vi "Debug Cell Performance.vi"() -> ()   [LabVIEW 2021]
uses:
  Ethernet/Ethernet_BS1201.lvclass
  TypeDefs/System Status.ctl
  BS120x.lvclass
panel:
  in  "Cell to view":i32=1 min=1 max=12
  out "I pk-pk 2":dbl
  out "I read average 2":dbl
  out "V pk-pk 2":dbl
  out "V Read Average 2":dbl
  in  "Run":bool
  in  "Number of Samples":i32=1 min=1 max=12
  in  "Precision":bool
  in  "PID Disable":bool
  in  "Reset Unit":bool
  out "error out":errorcluster
  out "Cell Current":dbl[](array[numeric]) format="%#8.1f"
  out "Cell Voltages":dbl[](array[numeric])
  in  "Voltage Set All":dbl
  in  "Sink I All":dbl
  in  "Source I All":dbl
  out "Status":T1
  in  "Enable All Cells":bool
  in  "UDP port":u16=54321
  in  "TCP port":u16=12345
  in  "Box IP address":string="192.168.1.100"
  in  "stop":bool
  out "Voltages 2":dbl[](graph)
  out "Currents 2":dbl[](graph)
  # "(c) 2019 Bloomy Controls, Inc. All rights reserved."
  # "Cell Performance"
  # "Configuration"
  # "Write All Channels"
  # "Read"
  # "1"
  # "6"
  # "Operational Config"
  # "12"
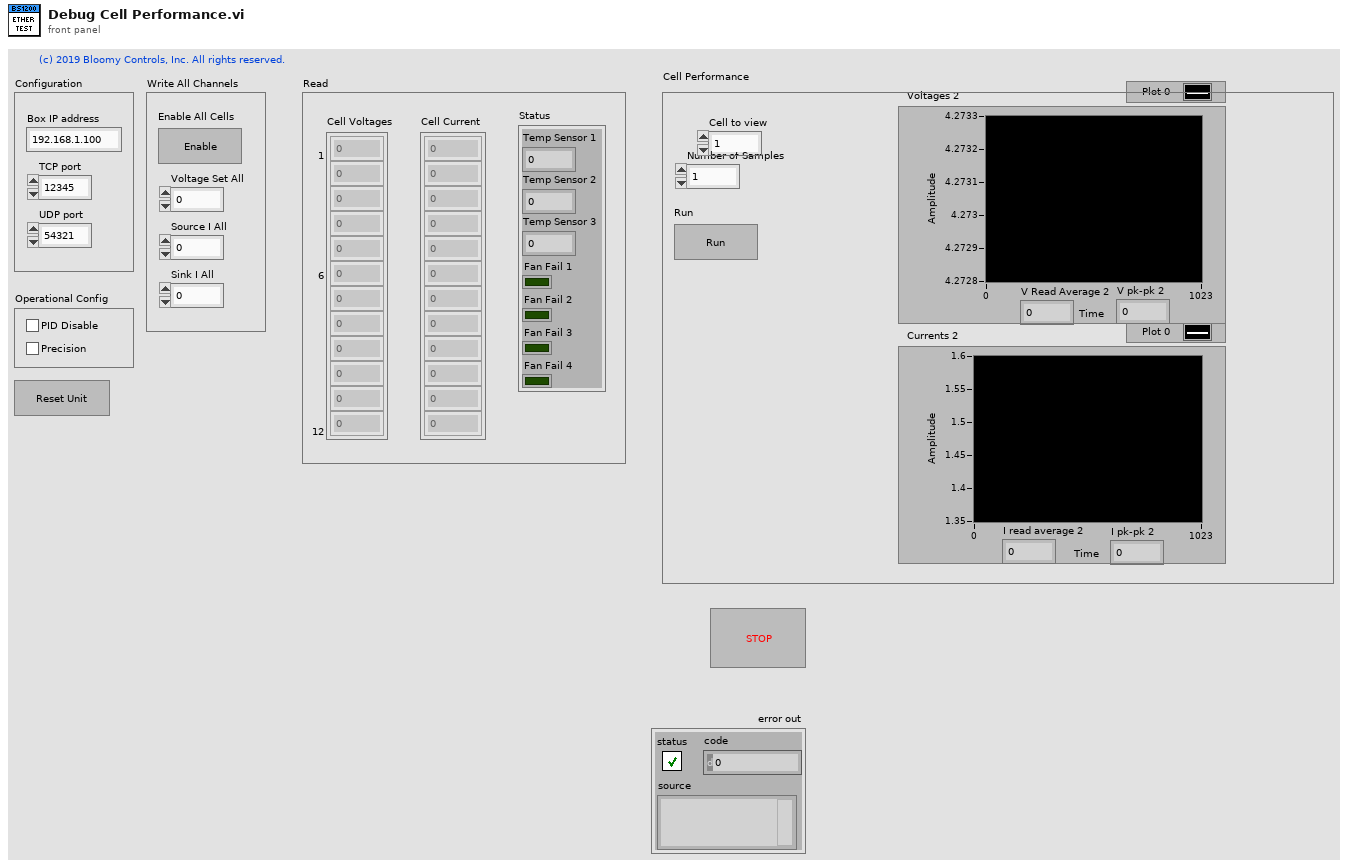
[diagram p1: front panel]
types:
  T1 = typedef "BS120x Driver.lvlib/BS120x.lvclass/System Status.ctl" = cluster{"Temp Sensor 1":dbl, "Temp Sensor 2":dbl, "Temp Sensor 3":dbl, "Fan Fail 1":bool, "Fan Fail 2":bool, "Fan Fail 3":bool, "Fan Fail 4":bool}
  T2 = typedef "Battery Simulator 1200 LabVIEW Driver.lvlib/Battery Simulator 1200 Driver.lvclass/System Status.ctl" = cluster{"Temp Sensor 1":dbl, "Temp Sensor 2":dbl, "Temp Sensor 3":dbl, "Fan Fail 1":bool, "Fan Fail 2":bool, "Fan Fail 3":bool, "Fan Fail 4":bool}
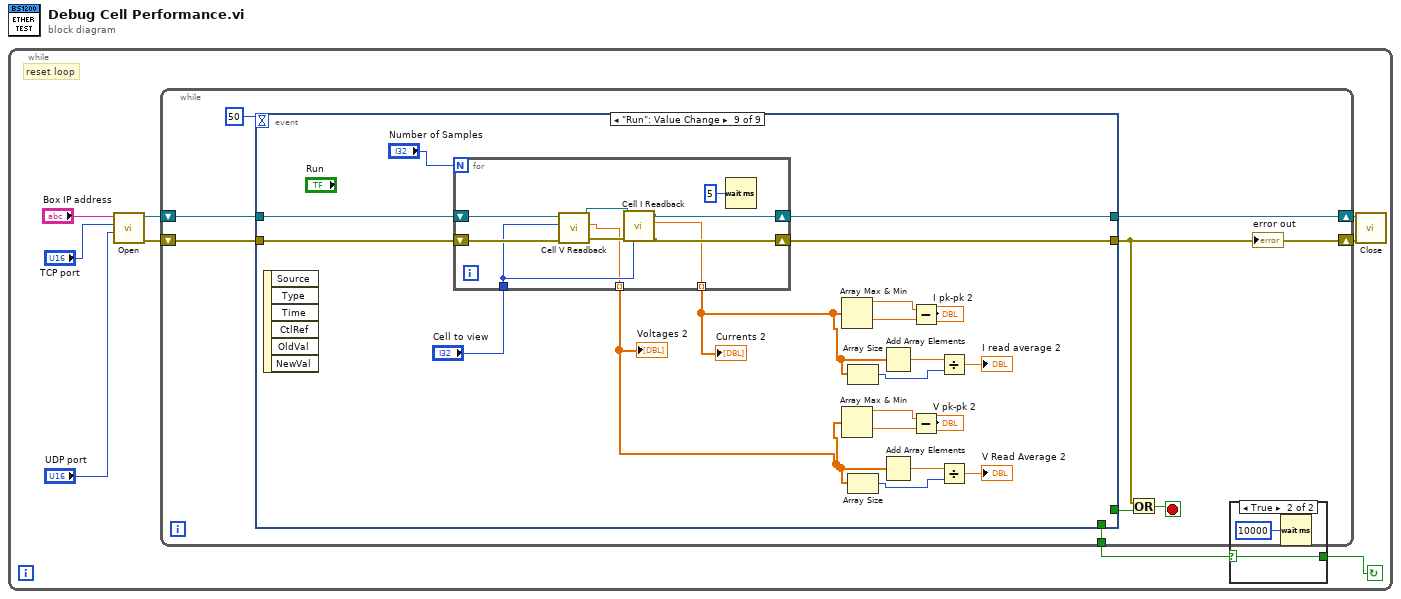
[diagram p0: block diagram]
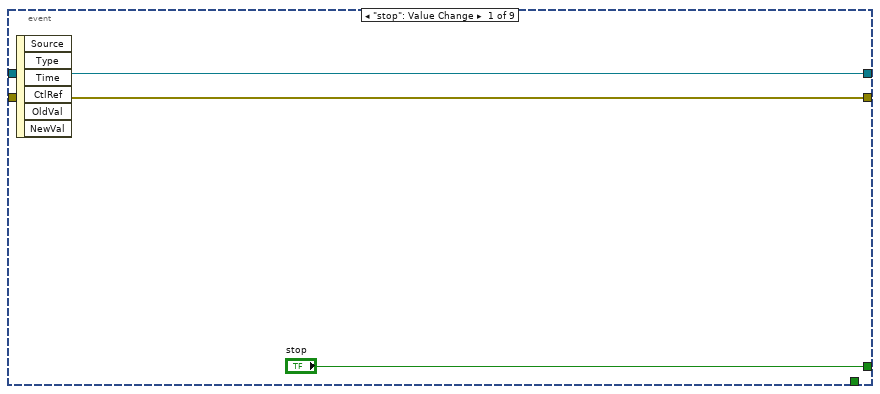
[diagram p3: hidden frame]
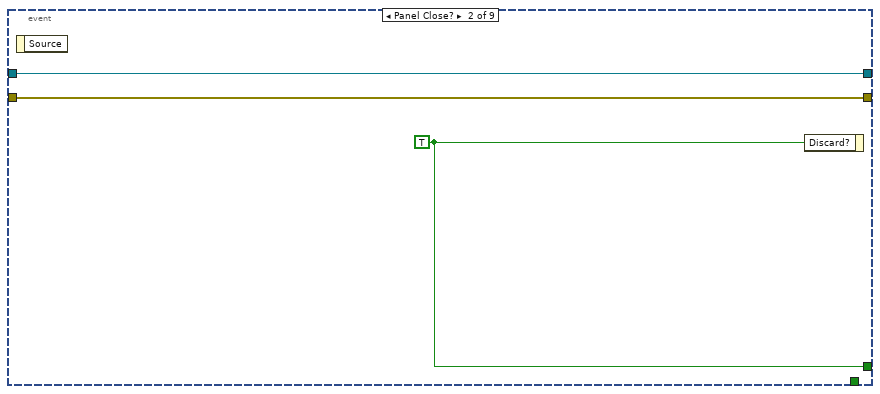
[diagram p4: hidden frame]
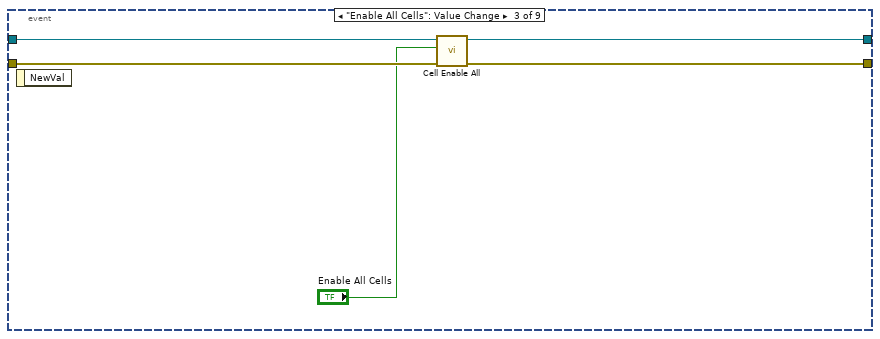
[diagram p5: hidden frame]
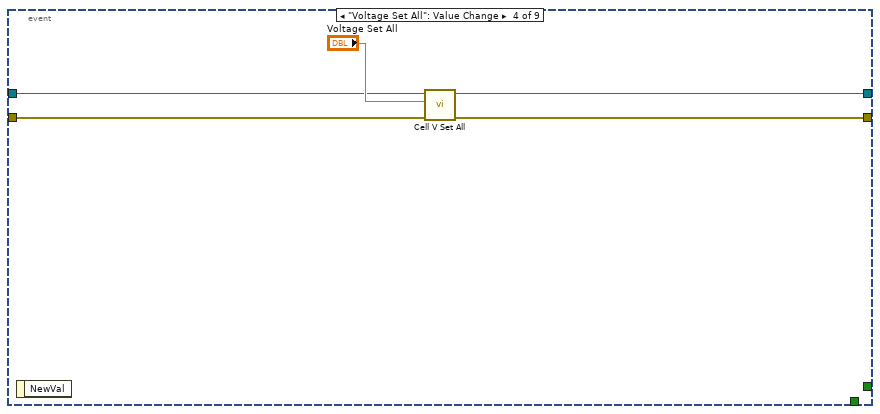
[diagram p6: hidden frame]
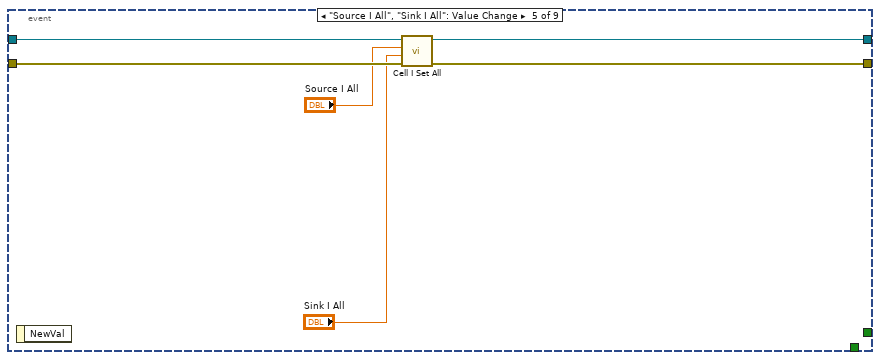
[diagram p7: hidden frame]
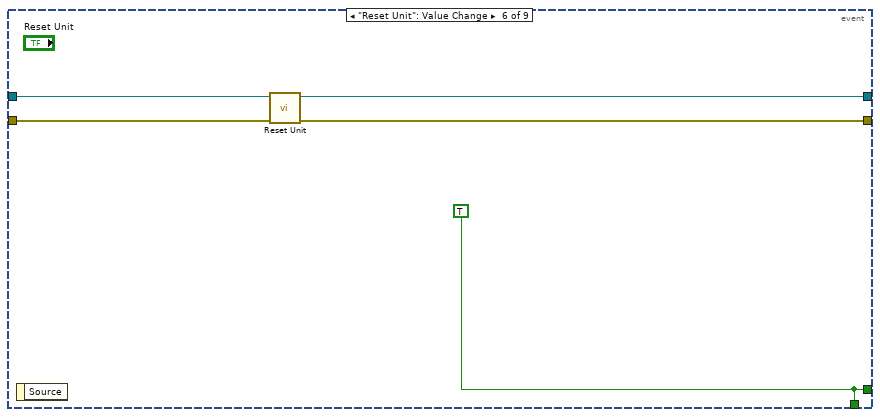
[diagram p8: hidden frame]
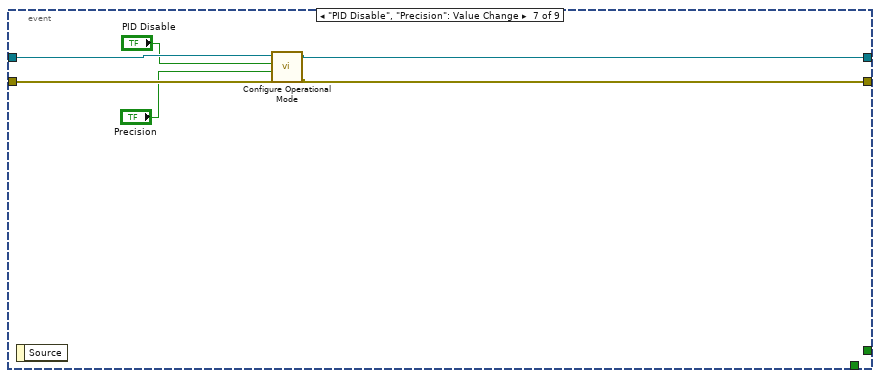
[diagram p9: hidden frame]
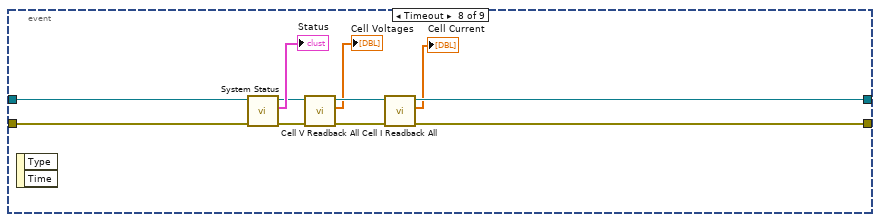
[diagram p10: hidden frame]
diagram:
  n1 = while {
    stop <- w1 continue-if-true
    # "reset loop"
    n2 = call "Open.vi"("UDP port"="UDP port", "TCP port"="TCP port", "Box IP address"="Box IP address") -> ("error out"=w3:errorcluster, "ENET out"=w7:refnum<class "Ethernet_BS1201.lvclass">)  [unwired: 7 in]
    n3 = while {
      shift-right: [w14] -> w10
      shift-left: w3 -> [w18]
      shift-right: [w20] -> w9
      shift-left: w7 -> [w19]
      tunnel: [w13] -> w2
      stop <- w16 stop-if-true
      n4 = event shown="[8] \"Run\": Value Change" {
        selector: _ -> [_ _ _ _ _ _ _ _ _]
        dyn-events: _ -> [_ _ _ _ _ _ _ _ _]
        timeout: 50 -> [_ _ _ _ _ _ _ _ _]
        tunnel: [w23 w26 w28 w32 w39 w46 w50 w63 w69] -> w20
        tunnel: w19 -> [w23 w26 w31 w35 w42 w47 w51 w54 w72]
        tunnel: [w22 w24 w27 w33 w40 w45 w52 w62 w68] -> w14
        tunnel: w18 -> [w22 w24 w30 w34 w41 w44 w53 w55 w71]
        tunnel: ["stop" w25 _ _ _ w43 _ _ _] -> w15
        tunnel: [_ _ _ _ _ w43 _ _ _] -> w13
        event "stop": Value Change {
          n5 = event-data() -> ()  [unwired: 1 in, 6 out]
        }
        event Panel Close? {
          w25 = TRUE ("Discard?")
          n6 = event-data() -> ()  [unwired: 1 in, 1 out]
          n7 = event-data("Discard?"=w25) -> ()  [unwired: 1 in, 1 out]
        }
        event "Enable All Cells": Value Change {
          n8 = event-data() -> ()  [unwired: 1 in, 1 out]
          n9 = call-dynamic "Cell Enable All.vi"("error in (no error)"=w30, "Enable"="Enable All Cells", "ENET in"=w31) -> ("error out"=w27:errorcluster, "ENET out"=w28:refnum<class "Ethernet_BS1201.lvclass">)  [unwired: 7 in]
        }
        event "Voltage Set All": Value Change {
          n10 = event-data() -> ()  [unwired: 1 in, 1 out]
          n11 = call-dynamic "Cell V Set All.vi"("error in (no error)"=w34, "Voltage"="Voltage Set All", "ENET in"=w35) -> ("error out"=w33:errorcluster, "ENET out"=w32:refnum<class "Ethernet_BS1201.lvclass">)  [unwired: 7 in]
        }
        event "Source I All", "Sink I All": Value Change {
          n12 = event-data() -> ()  [unwired: 1 in, 1 out]
          n13 = call-dynamic "Cell I Set All.vi"("error in (no error)"=w41, "Sink I All"="Sink I All", "Source I All"="Source I All", "ENET in"=w42) -> ("error out"=w40:errorcluster, "ENET out"=w39:refnum<class "Ethernet_BS1201.lvclass">)  [unwired: 6 in]
        }
        event "Reset Unit": Value Change {
          w43 = TRUE ("Discard?")
          n14 = event-data() -> ()  [unwired: 1 in, 1 out]
          n15 = call-dynamic "Reset Unit.vi"("error in (no error)"=w44, "Ethernet in"=w47) -> ("error out"=w45:errorcluster, "Ethernet out"=w46:refnum<class "Ethernet_BS1201.lvclass">)  [unwired: 8 in]
        }
        event "PID Disable", "Precision": Value Change {
          n16 = event-data() -> ()  [unwired: 1 in, 1 out]
          n17 = call-dynamic "Configure Operational Mode.vi"("error in (no error)"=w53, "Precision Mode"="Precision", "PID Disable"="PID Disable", "Ethernet in"=w51) -> ("error out"=w52:errorcluster, "Ethernet out"=w50:refnum<class "Ethernet_BS1201.lvclass">)  [unwired: 6 in]
        }
        event Timeout {
          n18 = event-data() -> ()  [unwired: 1 in, 2 out]
          n19 = call-dynamic "System Status.vi"("error in (no error)"=w55, "ENET in"=w54) -> ("error out"=w58:errorcluster, "Status"=→"Status":T2, "ENET out"=w60:refnum<class "Ethernet_BS1201.lvclass">)  [unwired: 7 in]
          n20 = call-dynamic "Cell V Readback All.vi"("error in (no error)"=w58, "ENET in"=w60) -> ("error out"=w59:errorcluster, "Voltage"=→"Cell Voltages":dbl[], "ENET out"=w61:refnum<class "Ethernet_BS1201.lvclass">)  [unwired: 7 in]
          n21 = call-dynamic "Cell I Readback All.vi"("error in (no error)"=w59, "ENET in"=w61) -> ("error out"=w62:errorcluster, "Current"=→"Cell Current":dbl[], "ENET out"=w63:refnum<class "Ethernet_BS1201.lvclass">)  [unwired: 7 in]
        }
        event "Run": Value Change {
          n22 = event-data() -> ()  [unwired: 1 in, 6 out]
          n23 = for {
            N: "Number of Samples" -> [_]
            tunnel: "Cell to view" -> [w90]
            shift-right: [w89] -> w69
            shift-left: w72 -> [w94]
            shift-right: [w88] -> w68
            shift-left: w71 -> [w93]
            tunnel: [w87] -> w66 mode=indexing
            tunnel: [w86] -> w67 mode=indexing
            n24 = call-dynamic "Cell V Readback.vi"("error in (no error)"=w93, "Channel"=w90, "ENET in"=w94) -> ("error out"=w91:errorcluster, "Voltage"=w87:dbl, "ENET out"=w92:refnum<class "Ethernet_BS1201.lvclass">)  [unwired: 6 in]
            n25 = call-dynamic "Cell I Readback.vi"("error in (no error)"=w91, "Channel"=w90, "ENET in"=w92) -> ("error out"=w88:errorcluster, "Current (mA)"=w86:dbl, "ENET out"=w89:refnum<class "Ethernet_BS1201.lvclass">)  [unwired: 6 in]
            n26 = Wait (ms)(milliseconds to wait=u32 5) -> ()  [unwired: 1 out]
          }
          "Voltages 2" <- w66
          "Currents 2" <- w67
          n27 = Array Max & Min(array=w67) -> (max value=w82:dbl, min value=w83:dbl)  [unwired: 2 out]
          n28 = Array Max & Min(array=w66) -> (max value=w76:dbl, min value=w75:dbl)  [unwired: 2 out]
          n29 = Array Size(array=w67) -> (size(s)=w79:i32)
          n30 = Array Size(array=w66) -> (size(s)=w73:i32)
          n31 = Add Array Elements(numeric array=w67) -> (sum=w81:dbl)
          n32 = Add Array Elements(numeric array=w66) -> (sum=w77:dbl)
          n33 = Subtract(x=w82, y=w83) -> (x-y=→"I pk-pk 2":dbl)
          n34 = Subtract(x=w76, y=w75) -> (x-y=→"V pk-pk 2":dbl)
          n35 = Divide(x=w81, y=w79) -> (x/y=→"I read average 2":dbl)
          n36 = Divide(x=w77, y=w73) -> (x/y=→"V Read Average 2":dbl)
        }
      }
      n37 = Or(x=w14, y=w15) -> (x .or. y?=w16:bool)
    }
    n38 = case shown="True" w2 {
      selector: w2 -> [_ w11]
      tunnel: [_ w11] -> w1
      frame False {
      }
      frame True {
        n39 = Wait (ms)(milliseconds to wait=u32 10000) -> ()  [unwired: 1 out]
      }
    }
    n40 = call-dynamic "Close.vi"("error in (no error)"=w10, "ENET in"=w9) -> ("error out"=→"error out":errorcluster)  [unwired: 9 in]
  }
